vi "varXNode_GenerateCode.vi"(1 "Terms":cluster{"Term":refnum<vi>, "ID":string}[](array[cluster]), 3 "Diagram":refnum<vi>, 5 "XRef":refnum<vi>, 6 "State In":T1) -> (0 "Generated Code?":bool, 2 "State Out":T1, 4 "Reply":string[](array[string]))   [LabVIEW 2017, in "varXNode.xnode"]
uses:
  <vilib>/variable/varXNode.llb/varXNode.xnode
  <vilib>/variable/varXNode.llb/varXNode.ctl
  <vilib>/variable/Type Descriptor.ctl
  <vilib>/variable/NI_Variable.lvlib
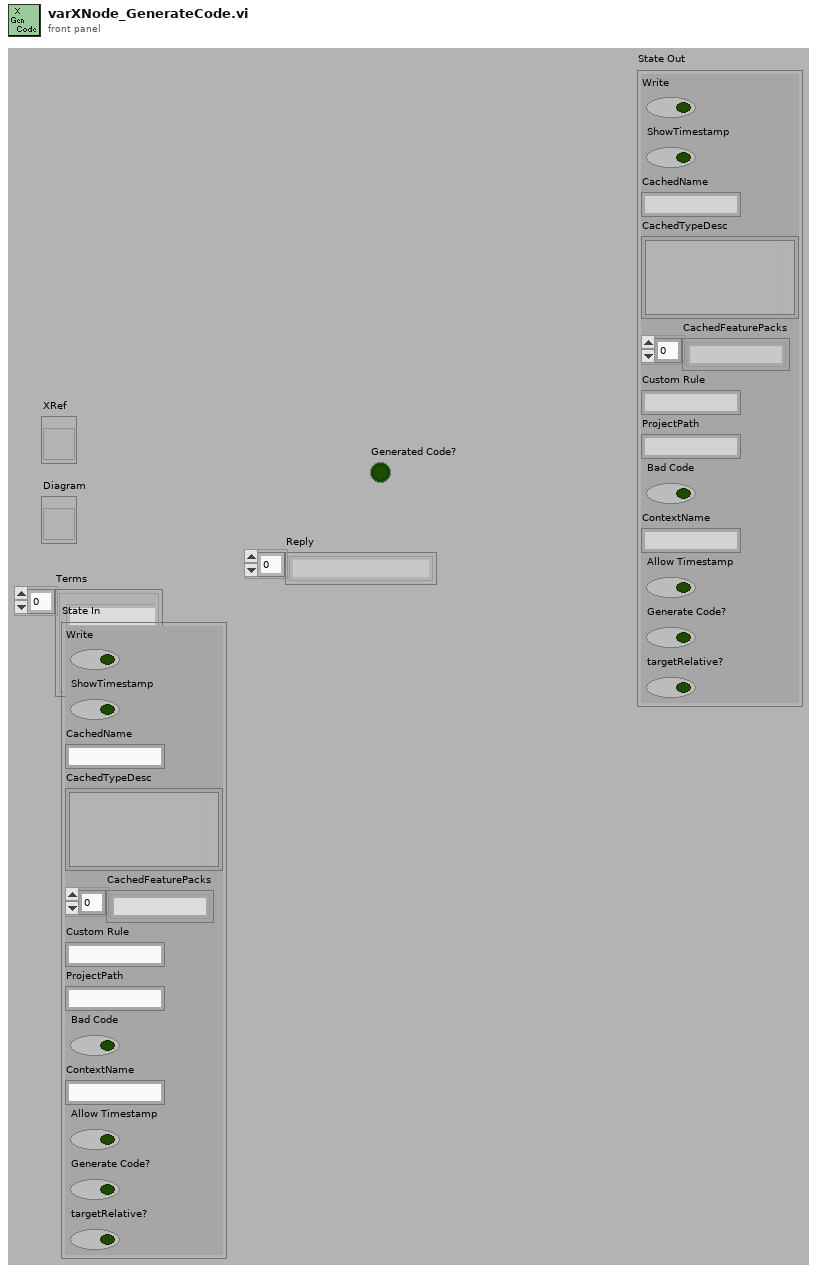
[diagram p1: front panel]
types:
  T1 = typedef "varXNode.xnode/varXNode.ctl" = cluster{"Write":bool, "ShowTimestamp":bool, "CachedName":string, "CachedTypeDesc":T2, "CachedFeaturePacks":string[], "Custom Rule":string, "ProjectPath":string, "Bad Code":bool, "ContextName":string, "Allow Timestamp":bool, "Generate Code?":bool, "targetRelative?":bool}
  T2 = typedef "NI_Variable.lvlib/Type Descriptor.ctl" = cluster{"Variant":variant}
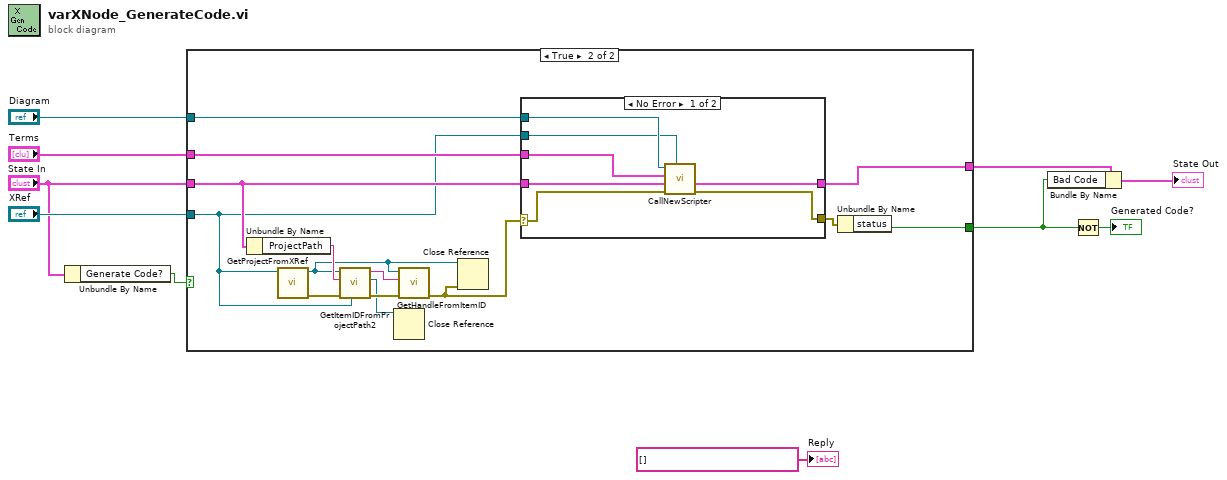
[diagram p0: block diagram]
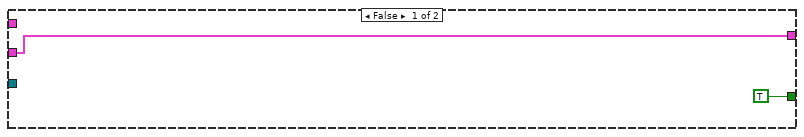
[diagram p2: hidden frame]
diagram:
  n1 = Unbundle By Name("State In") -> ("Generate Code?"=w1:bool)
  n2 = case shown="True" w1 {
    tunnel: "Diagram" -> [_ w26]
    tunnel: "Terms" -> [_ w25]
    tunnel: "State In" -> [w12 w24]
    tunnel: "XRef" -> [_ w13]
    tunnel: [w12 w15] -> w4
    tunnel: [TRUE ("status") w14] -> w3
    frame False {
    }
    frame True {
      n3 = Unbundle By Name(w24) -> ("ProjectPath"=w20:string)
      n4 = call <vilib>:"GetProjectFromXRef.vi"("XRef"=w13) -> ("error out"=w23:errorcluster, "Project"=w19:refnum<vi>)  [unwired: 9 in]
      n5 = call <vilib>:"GetItemIDFromProjectPath2.vi"("XRef"=w13, "error in"=w23, "ProjectPath"=w20, "Project"=w19) -> ("error out"=w22:errorcluster, "ProjectItem"=w17:refnum<vi>, "Item ID"=w21:string)  [unwired: 5 in]
      n6 = Close Reference(reference=w17) -> ()  [unwired: 1 in, 1 out]
      n7 = call <vilib>:"GetHandleFromItemID.vi"("error in"=w22, "ItemID"=w21, "Project"=w19) -> ("error out"=w18:errorcluster)  [unwired: 7 in, 1 out]
      n8 = Close Reference(reference=w19, error in (no error)=w18) -> ()  [unwired: 1 out]
      n9 = case shown="No Error" w18 {
        selector: w18 -> [w28 w34]
        tunnel: w26 -> [w33 _]
        tunnel: w25 -> [w32 _]
        tunnel: w24 -> [w31 w35]
        tunnel: [w30 w35] -> w15
        tunnel: [w27 w34] -> w16
        tunnel: w13 -> [w29 _]
        frame No Error {
          n10 = call <vilib>:"CallNewScripter.vi"("XRef"=w29, "error in"=w28, "State In"=w31, "Terms"=w32, "Diagram"=w33) -> ("error out"=w27:errorcluster, "State Out"=w30:T1)  [unwired: 5 in]
        }
        frame Error {
        }
      }
      n11 = Unbundle By Name(w16) -> ("status"=w14:bool)
    }
  }
  n12 = Bundle By Name(cluster=w4, "Bad Code"=w3) -> (→"State Out":T1)
  n13 = Not(x=w3) -> (.not. x?=→"Generated Code?":bool)
  "Reply" <- string[] [] ("Reply")
